vi "DI-Off-Delay.vi"(10 "Count":i32=10000, 11 "Boolean-01":bool) -> (2 "Boolean-01 Count":i32, 3 "Boolean-01-Indicator":bool)   [LabVIEW 2015]
panel:
  out "Numeric":i32
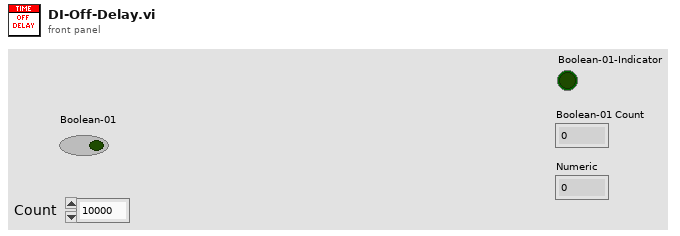
[diagram p1: front panel]
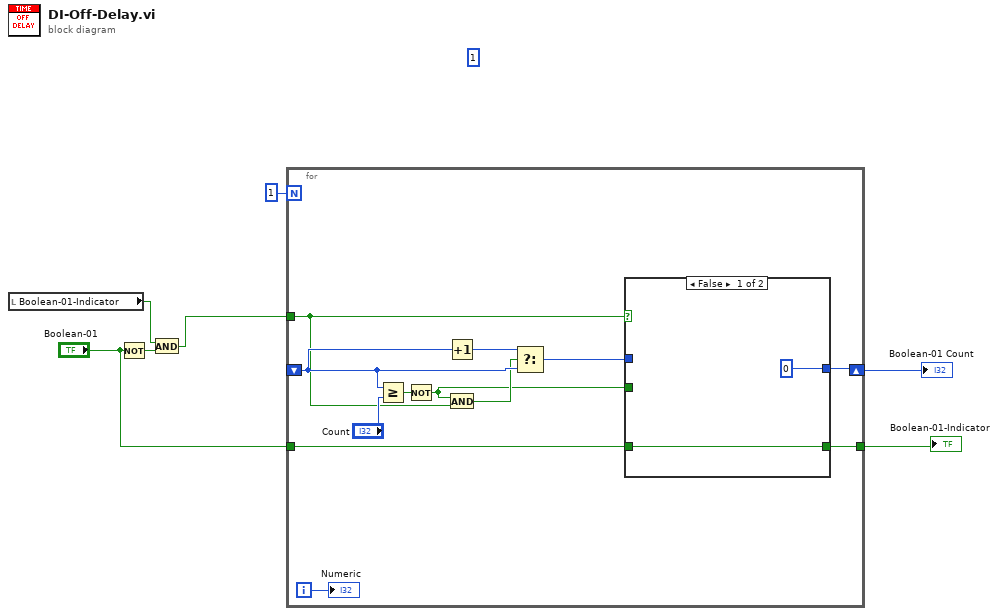
[diagram p0: block diagram]
diagram:
  (unwired) 1
  n1 = local read "Boolean-01-Indicator"() -> (w7:bool)
  n2 = Not(x="Boolean-01") -> (.not. x?=w6:bool)
  n3 = And(x=w7, y=w6) -> (x .and. y?=w4:bool)
  n4 = for {
    N: 1 -> [_]
    shift-right: [w15] -> w3
    shift-left: _ -> [w12]
    tunnel: w4 -> [w10]
    tunnel: "Boolean-01" -> [w14]
    tunnel: [w13] -> w1
    i -> [w17]
    n5 = Greater Or Equal?(x=w12, y="Count") -> (x >= y?=w11:bool)
    n6 = Not(x=w11) -> (.not. x?=w8:bool)
    n7 = Increment(x=w12) -> (x+1=w19:i32)
    n8 = And(x=w8, y=w10) -> (x .and. y?=w9:bool)
    n9 = Select(t=w19, s=w9, f=w12) -> (s? t:f=w16:i32)
    n10 = case shown="False" w10 {
      tunnel: w16 -> [_ w23]
      tunnel: [0 ("Boolean-01 Count") w23] -> w15
      tunnel: w14 -> [w20 _]
      tunnel: [w20 w22] -> w13
      tunnel: w8 -> [_ w22]
      frame False {
      }
      frame True {
      }
    }
    "Numeric" <- w17
  }
  "Boolean-01-Indicator" <- w1
  "Boolean-01 Count" <- w3
